vi "ConfigUtilities - Initialize Device Sections and Channels.vi"(8 "error in (no error)":errorcluster, 11 "Item Ref out":T1 format="%.0x") -> (0 "error out":errorcluster, 3 "Parent Ref out":T1 format="%.0x")   [LabVIEW 2016, in "UDP-Custom-Device System Explorer.lvlib"]
doc: "Add Status Channels and Receive (Rx) Channels Section to the system definition."
uses:
  UDP-Custom-Device System Explorer.lvlib
  <vilib>/NI Veristand/Custom Device API/Custom Device Item Ref.ctl
  Shared/Constants.vi
  <vilib>/NI VeriStand/Custom Device API/Custom Device API.lvlib
  <vilib>/NI Veristand/Custom Device API/Custom Device Channel Type.ctl
  <vilib>/NI Veristand/Custom Device API/Custom Device Channel.ctl
  Shared/UDP-Custom-Device Shared.lvlib
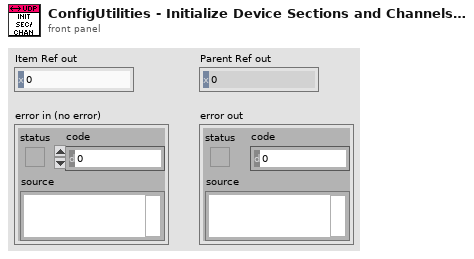
[diagram p1: front panel]
types:
  T1 = typedef "Custom Device API.lvlib/Custom Device Item Ref.ctl" = u64
  T2 = typedef "Custom Device API.lvlib/Custom Device Channel.ctl" = cluster{"Type":T3, "Units":string, "Default Value":dbl, "Faultable":bool, "Scalable":bool}
  T3 = typedef "Custom Device API.lvlib/Custom Device Channel Type.ctl" = enum16{"Input", "Output"}
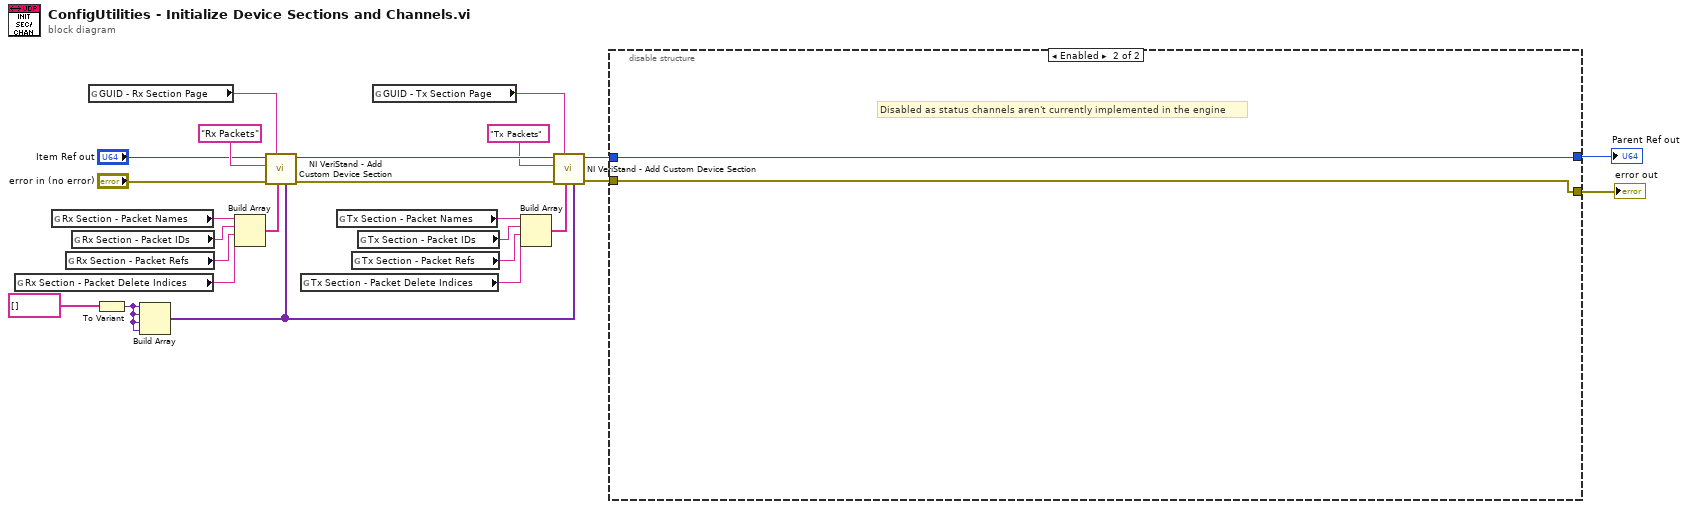
[diagram p0: block diagram]
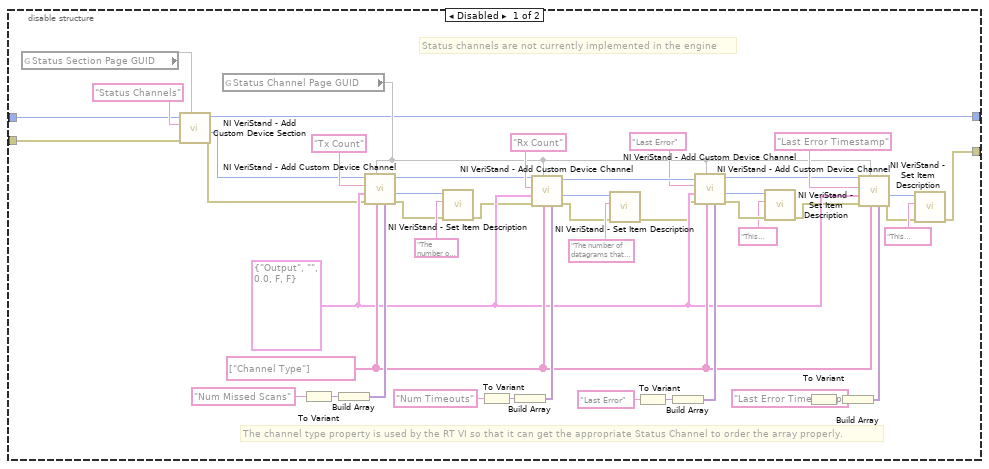
[diagram p2: hidden frame]
diagram:
  n1 = global read "Constants.vi" "Rx Section - Packet Delete Indices"() -> (w13:string)
  n2 = global read "Constants.vi" "Rx Section - Packet Names"() -> (w15:string)
  n3 = global read "Constants.vi" "Rx Section - Packet Refs"() -> (w12:string)
  n4 = global read "Constants.vi" "Rx Section - Packet IDs"() -> (w14:string)
  n5 = global read "Constants.vi" "GUID - Rx Section Page"() -> (w17:string)
  n6 = To Variant(anything=string[] []) -> (Variant=w18:variant)
  n7 = Build Array(w18, w18, w18, w18) -> (w19:variant[])
  n8 = Build Array(w15, w14, w12, w13) -> (w20:string[])
  n9 = call <vilib>:"NI VeriStand - Add Custom Device Section.vi"("Property Values"=w19, "Property names"=w20, "GUID (Default Section)"=w17, "error in (no error)"="error in (no error)", "Section Name"="Rx Packets", "Parent Ref in"="Item Ref out") -> ("error out"=w23:errorcluster, "Parent Ref out"=w24:T1)  [unwired: 2 in, 2 out]
  n10 = global read "Constants.vi" "Tx Section - Packet Delete Indices"() -> (w10:string)
  n11 = global read "Constants.vi" "Tx Section - Packet Names"() -> (w8:string)
  n12 = global read "Constants.vi" "Tx Section - Packet Refs"() -> (w11:string)
  n13 = global read "Constants.vi" "Tx Section - Packet IDs"() -> (w9:string)
  n14 = global read "Constants.vi" "GUID - Tx Section Page"() -> (w16:string)
  n15 = Build Array(w8, w9, w11, w10) -> (w7:string[])
  n16 = call <vilib>:"NI VeriStand - Add Custom Device Section.vi"("Property Values"=w19, "Property names"=w7, "GUID (Default Section)"=w16, "error in (no error)"=w23, "Section Name"="Tx Packets", "Parent Ref in"=w24) -> ("error out"=w5:errorcluster, "Parent Ref out"=w6:T1)  [unwired: 2 in, 2 out]
  n17 = disable-structure shown="Enabled" {
    disable-tunnel: w6 -> [w30 w72]
    disable-tunnel: w5 -> [w29 w71]
    disable-tunnel: [w28 w71] -> w2
    disable-tunnel: [w27 w72] -> w1
    frame Disabled {
      w58 = string[] ["Channel Type"] ("Property names")
      w57 = T2 {"Type"=enum."Output", "Units"="", "Default Value"=0.0, "Faultable"=FALSE, "Scalable"=FALSE} ("Channel")
      # "Status channels are not currently implemented in the engine"
      # "The channel type property is used by the RT VI so that it can get the appropriate Status Channel to order the array properly."
      n18 = global read "Constants.vi" "Status Section Page GUID"() -> (w31)
      n19 = call <vilib>:"NI VeriStand - Add Custom Device Section.vi"("GUID (Default Section)"=w31, "error in (no error)"=w29, "Section Name"="Status Channels", "Parent Ref in"=w30) -> ("error out"=w47:errorcluster, "Section Ptr"=w26:T1, "Parent Ref out"=w27:T1)  [unwired: 4 in, 1 out]
      n20 = global read "Constants.vi" "Status Channel Page GUID"() -> (w32)
      n21 = To Variant(anything="Num Missed Scans" ("String")) -> (Variant=w60:variant)
      n22 = Build Array(w60) -> (w61:variant[])
      n23 = call <vilib>:"NI VeriStand - Add Custom Device Channel.vi"("Property Values"=w61, "Property names"=w58, "GUID (Default Channel)"=w32, "error in (no error)"=w47, "Channel"=w57, "Channel Name"="Tx Count", "Parent Ref in"=w26) -> ("error out"=w45:errorcluster, "Channel Ref"=w46:T1, "Parent Ref out"=w51:T1)  [unwired: 1 in, 1 out]
      n24 = call <vilib>:"NI VeriStand - Set Item Description.vi"("error in (no error)"=w45, "Description"="The number of datagrams that have not been transmitted.", "Item Ref in"=w46) -> ("error out"=w53:errorcluster)  [unwired: 6 in, 2 out]
      n25 = To Variant(anything="Num Timeouts" ("String")) -> (Variant=w62:variant)
      n26 = Build Array(w62) -> (w64:variant[])
      n27 = call <vilib>:"NI VeriStand - Add Custom Device Channel.vi"("Property Values"=w64, "Property names"=w58, "GUID (Default Channel)"=w32, "error in (no error)"=w53, "Channel"=w57, "Channel Name"="Rx Count", "Parent Ref in"=w51) -> ("error out"=w50:errorcluster, "Channel Ref"=w49:T1, "Parent Ref out"=w52:T1)  [unwired: 1 in, 1 out]
      n28 = call <vilib>:"NI VeriStand - Set Item Description.vi"("error in (no error)"=w50, "Description"="The number of datagrams that have not been received.", "Item Ref in"=w49) -> ("error out"=w54:errorcluster)  [unwired: 6 in, 2 out]
      n29 = To Variant(anything="Last Error" ("String")) -> (Variant=w66:variant)
      n30 = Build Array(w66) -> (w67:variant[])
      n31 = call <vilib>:"NI VeriStand - Add Custom Device Channel.vi"("Property Values"=w67, "Property names"=w58, "GUID (Default Channel)"=w32, "error in (no error)"=w54, "Channel"=w57, "Channel Name"="Last Error", "Parent Ref in"=w52) -> ("error out"=w41:errorcluster, "Channel Ref"=w35:T1, "Parent Ref out"=w33:T1)  [unwired: 1 in, 1 out]
      n32 = call <vilib>:"NI VeriStand - Set Item Description.vi"("error in (no error)"=w41, "Description"="This Channel gives the last error of TCP Server. There is no distinction between error and warning.", "Item Ref in"=w35) -> ("error out"=w36:errorcluster)  [unwired: 6 in, 2 out]
      n33 = To Variant(anything="Last Error Timestamp" ("String")) -> (Variant=w68:variant)
      n34 = Build Array(w68) -> (w70:variant[])
      n35 = call <vilib>:"NI VeriStand - Add Custom Device Channel.vi"("Property Values"=w70, "Property names"=w58, "GUID (Default Channel)"=w32, "error in (no error)"=w36, "Channel"=w57, "Channel Name"="Last Error Timestamp", "Parent Ref in"=w33) -> ("error out"=w38:errorcluster, "Channel Ref"=w34:T1)  [unwired: 1 in, 2 out]
      n36 = call <vilib>:"NI VeriStand - Set Item Description.vi"("error in (no error)"=w38, "Description"="This Channel gives the System Time When the Channel \"Server Last Error\" was last updated.", "Item Ref in"=w34) -> ("error out"=w28:errorcluster)  [unwired: 6 in, 2 out]
    }
    frame Enabled {
      # "Disabled as status channels aren't currently implemented in the engine"
    }
  }
  "Parent Ref out" <- w1
  "error out" <- w2
